vi "Query Status.vi"(8 "error in":errorcluster, 11 "2727 in":refnum<class "2727.lvclass">) -> (0 "error out":errorcluster, 2 "Resistance":dbl[](array[numeric]), 3 "2727 out":refnum<class "2727.lvclass">)   [LabVIEW 2019, in "2727.lvlib" / "2727.lvclass"]
uses:
  Library/2727.lvclass
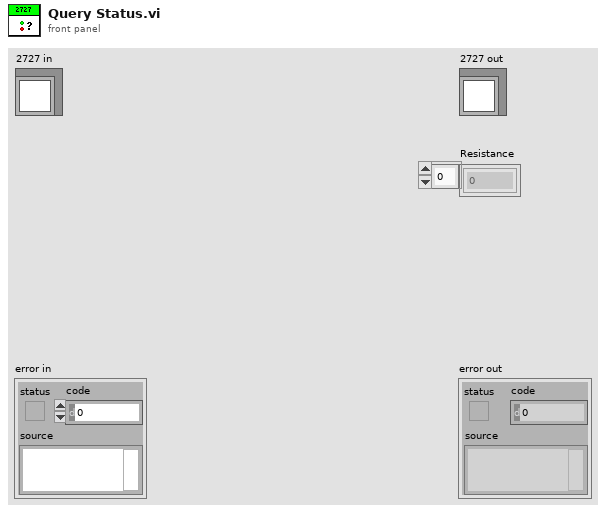
[diagram p1: front panel]
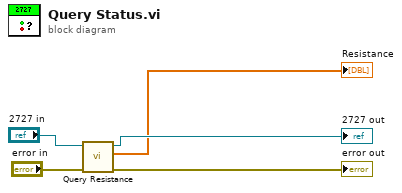
[diagram p0: block diagram]
diagram:
  n1 = call "Query Resistance.vi"("error in"="error in", "2727 in"="2727 in") -> ("error out"=→"error out":errorcluster, "Resistance"=→"Resistance":dbl[], "2727 out"=→"2727 out":refnum<class "2727.lvclass">)  [unwired: 7 in]
